vi "Decimate and add.vi"(7 "DAQ":T1={"Data"={"Live"={"t0"=timestamp(0 s since 1904-01-01), "dt"=1.0, "Y"=[]}, "Accumulated"={"t0"=timestamp(0 s since 1904-01-01), "dt"=1.0, "Y"=[]}, "Averaged"={"t0"=timestamp(0 s since 1904-01-01), "dt"=1.0, "Y"=[]}, "data array"=[], "live time array"=[], "Live (decimated)"={"t0"=timestamp(0 s since 1904-01-01), "dt"=1.0, "Y"=[]}}, "Config"={"Input Config"=0, "Card"=enum."USB-6211", "100% Reflectance Standard (V)"=0.0, "Input Channel"="", "Average number of points"=0.0, "Trigger Level (V)"=0.0, "Rate (Hz)"=0, "End Time (s)"=0.0}, "Indicators"={"Final number of points"=0.0, "Number of samples"=0.0, "dt"=0.0, "Shots"=10, "Shot counter"=10, "Test counter"=10, "Background level (V)"=0.0, "DAQ task"="", "timestamp of data"=timestamp(0 s since 1904-01-01), "Test Type"=enum."A-Test"}} {"Config"."Input Config" items=["default"=-1, "RSE"=10083, "NRSE"=10078, "Differential"=10106, "Pseudodifferential"=12529]}, 8 "error in":errorcluster) -> (0 "error out":errorcluster, 3 "Decimated live data":dbl[](graph), 5 "DAQ out":T1={"Data"={"Live"={"t0"=timestamp(0 s since 1904-01-01), "dt"=1.0, "Y"=[]}, "Accumulated"={"t0"=timestamp(0 s since 1904-01-01), "dt"=1.0, "Y"=[]}, "Averaged"={"t0"=timestamp(0 s since 1904-01-01), "dt"=1.0, "Y"=[]}, "data array"=[], "live time array"=[], "Live (decimated)"={"t0"=timestamp(0 s since 1904-01-01), "dt"=1.0, "Y"=[]}}, "Config"={"Input Config"=0, "Card"=enum."USB-6211", "100% Reflectance Standard (V)"=0.0, "Input Channel"="", "Average number of points"=0.0, "Trigger Level (V)"=0.0, "Rate (Hz)"=0, "End Time (s)"=0.0}, "Indicators"={"Final number of points"=0.0, "Number of samples"=0.0, "dt"=0.0, "Shots"=10, "Shot counter"=10, "Test counter"=10, "Background level (V)"=0.0, "DAQ task"="", "timestamp of data"=timestamp(0 s since 1904-01-01), "Test Type"=enum."A-Test"}} {"Config"."Input Config" items=["default"=-1, "RSE"=10083, "NRSE"=10078, "Differential"=10106, "Pseudodifferential"=12529]})   [LabVIEW 2017, in "DAQ.lvlib"]
uses:
  DAQ.lvlib
  Controls/Params.ctl
  Controls/DAQ Config.ctl
  Controls/DAQ Indicators.ctl
  System Control/CTLs/Test Type.ctl
  <vilib>/Analysis/2dsp.llb/Decimate (single shot, DBL).vi
  <vilib>/Analysis/NI_AALPro.lvlib
  System Control/Main controller.lvlib
panel:
  out "Waveform Graph 2":waveform(dbl)(graph)
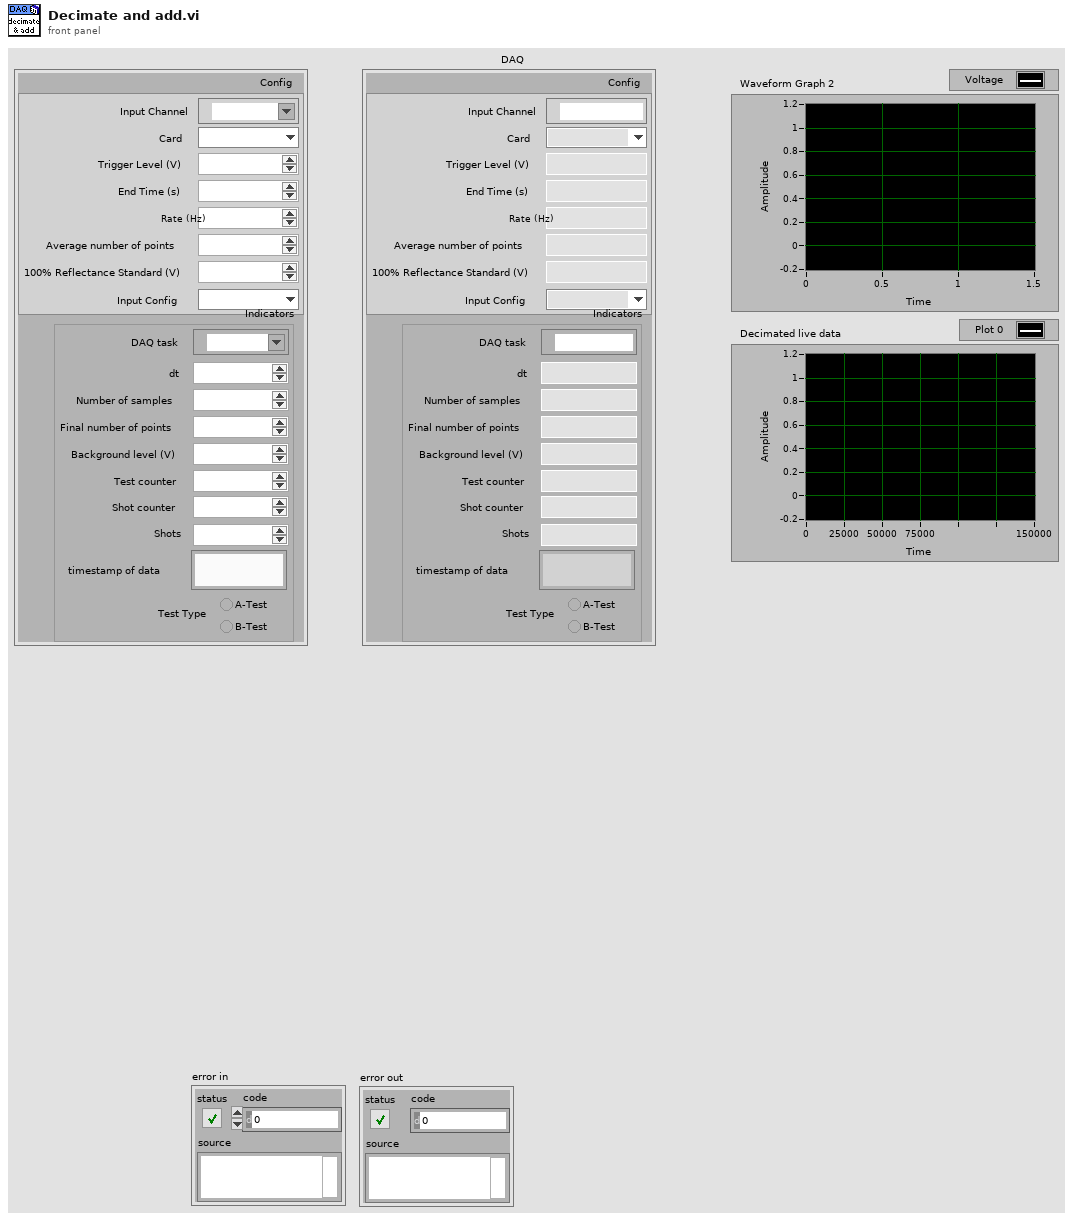
[diagram p1: front panel]
types:
  T1 = typedef "DAQ.lvlib/Params.ctl" = cluster{"Data":cluster{"Live":waveform(dbl), "Accumulated":waveform(dbl), "Averaged":waveform(dbl), "data array":dbl[], "live time array":dbl[], "Live (decimated)":waveform(dbl)}, "Config":T2, "Indicators":T3}
  T2 = typedef "DAQ.lvlib/DAQ Config.ctl" = cluster{"Input Config":i32, "Card":enum16{"USB-6211", "USB-6251", "USB-6361"}, "100% Reflectance Standard (V)":dbl, "Input Channel":tag, "Average number of points":dbl, "Trigger Level (V)":dbl, "Rate (Hz)":i32, "End Time (s)":dbl}
  T3 = typedef "DAQ.lvlib/DAQ Indicators.ctl" = cluster{"Final number of points":dbl, "Number of samples":dbl, "dt":dbl, "Shots":i32, "Shot counter":i32, "Test counter":i32, "Background level (V)":dbl, "DAQ task":refnum<k21>, "timestamp of data":timestamp, "Test Type":T4}
  T4 = typedef "Main controller.lvlib/Test Type.ctl" = enum32{"A-Test", "B-Test"}
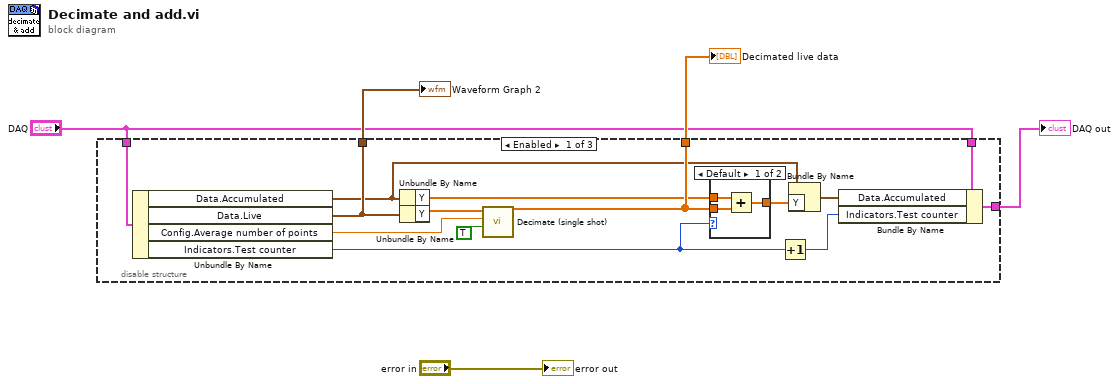
[diagram p0: block diagram]
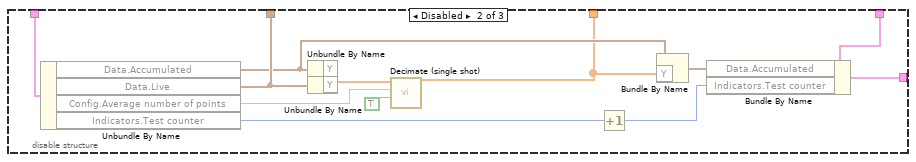
[diagram p3: hidden frame]
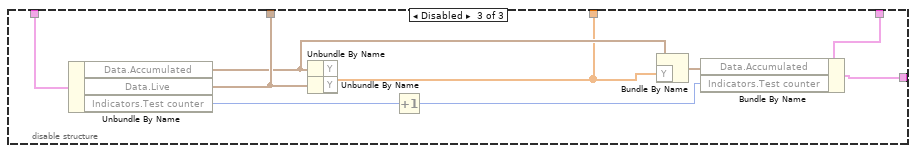
[diagram p4: hidden frame]
diagram:
  n1 = disable-structure shown="Enabled" {
    disable-tunnel: [w16 w32 w44] -> w4
    disable-tunnel: [w15 w24 w36] -> w3
    disable-tunnel: [w14 w31 w43] -> w2
    disable-tunnel: "DAQ" -> [w13 w30 w42]
    disable-tunnel: "DAQ" -> [w7 w25 w39]
    frame Enabled {
      n2 = Unbundle By Name(w7) -> ("Data.Accumulated"=w8:waveform(dbl), "Data.Live"=w14:waveform(dbl), "Config.Average number of points"=w19:dbl, "Indicators.Test counter"=w6:i32)
      n3 = Unbundle By Name(w8) -> ("Y"=w10:dbl[])
      n4 = Unbundle By Name(w14) -> ("Y"=w17:dbl[])
      n5 = call-poly <vilib>:"Decimate (single shot).vi"("averaging"=TRUE, "decimating factor"=w19, "X"=w17) -> ("Decimated Array"=w15:dbl[])  [unwired: 7 in, 1 out]
      n6 = case shown="Default" w6 {
        tunnel: w15 -> [w22 w23]
        tunnel: w10 -> [w21 _]
        tunnel: [w20 w23] -> w9
        frame Default {
          n7 = Add(x=w21, y=w22) -> (x+y=w20:dbl[])
        }
        frame 0 {
        }
      }
      n8 = Increment(x=w6) -> (x+1=w12:i32)
      n9 = Bundle By Name(cluster=w8, "Y"=w9) -> (w11:waveform(dbl))
      n10 = Bundle By Name(cluster=w13, "Data.Accumulated"=w11, "Indicators.Test counter"=w12) -> (w16:T1)
    }
    frame Disabled {
      n11 = Unbundle By Name(w25) -> ("Data.Accumulated"=w26:waveform(dbl), "Data.Live"=w31:waveform(dbl), "Config.Average number of points"=w35:dbl, "Indicators.Test counter"=w29:i32)
      n12 = Unbundle By Name(w26) -> ()  [unwired: 1 out]
      n13 = Unbundle By Name(w31) -> ("Y"=w33:dbl[])
      n14 = call-poly <vilib>:"Decimate (single shot).vi"("averaging"=TRUE, "decimating factor"=w35, "X"=w33) -> ("Decimated Array"=w24:dbl[])  [unwired: 7 in, 1 out]
      n15 = Increment(x=w29) -> (x+1=w28:i32)
      n16 = Bundle By Name(cluster=w26, "Y"=w24) -> (w27:waveform(dbl))
      n17 = Bundle By Name(cluster=w30, "Data.Accumulated"=w27, "Indicators.Test counter"=w28) -> (w32:T1)
    }
    frame Disabled {
      n18 = Unbundle By Name(w39) -> ("Data.Accumulated"=w40:waveform(dbl), "Data.Live"=w43:waveform(dbl), "Indicators.Test counter"=w38:i32)
      n19 = Unbundle By Name(w40) -> ()  [unwired: 1 out]
      n20 = Unbundle By Name(w43) -> ("Y"=w36:dbl[])
      n21 = Increment(x=w38) -> (x+1=w37:i32)
      n22 = Bundle By Name(cluster=w40, "Y"=w36) -> (w41:waveform(dbl))
      n23 = Bundle By Name(cluster=w42, "Data.Accumulated"=w41, "Indicators.Test counter"=w37) -> (w44:T1)
    }
  }
  "DAQ out" <- w4
  "Decimated live data" <- w3
  "Waveform Graph 2" <- w2
  "error out" <- "error in"
